vi "Testing FXP18-to-I16 conversions.vi"() -> ()   [LabVIEW 2015]
uses:
  <instrlib>/_niInstr/DSP/v1/Shared/Public/IQ Data.ctl
  DDC_7976R_v1.lvlib
  <vilib>/Analysis/NI_AALBase.lvlib
  <instrlib>/_niInstr/DSP/v1/Shared/niInstr DSP v1 Shared.lvlib
panel:
  out "appended array":dbl[][](graph)
  out "double precision float":dbl
  out "*(type *) &x":fxp<+/-,18,1> format="%.18g"
  out "Numeric Control":u32
  in  "data":T1
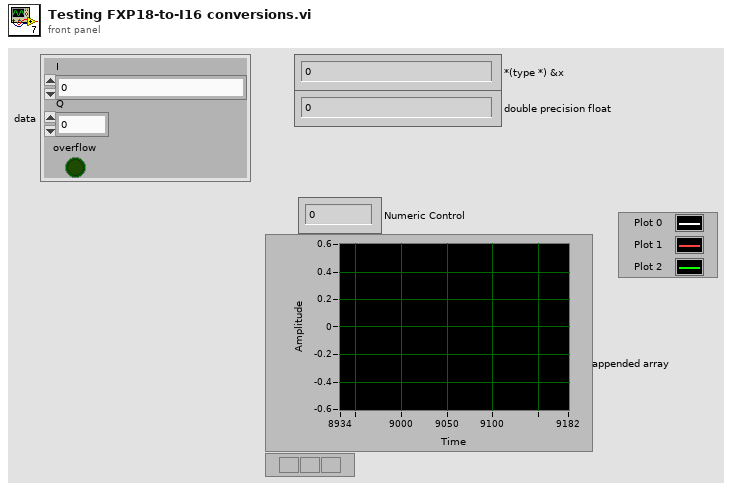
[diagram p1: front panel]
types:
  T1 = typedef "niInstr DSP v1 Shared.lvlib/IQ Data.ctl" = cluster{"I":fxp<+/-,18,1>, "Q":fxp<+/-,18,1>, "overflow":bool}
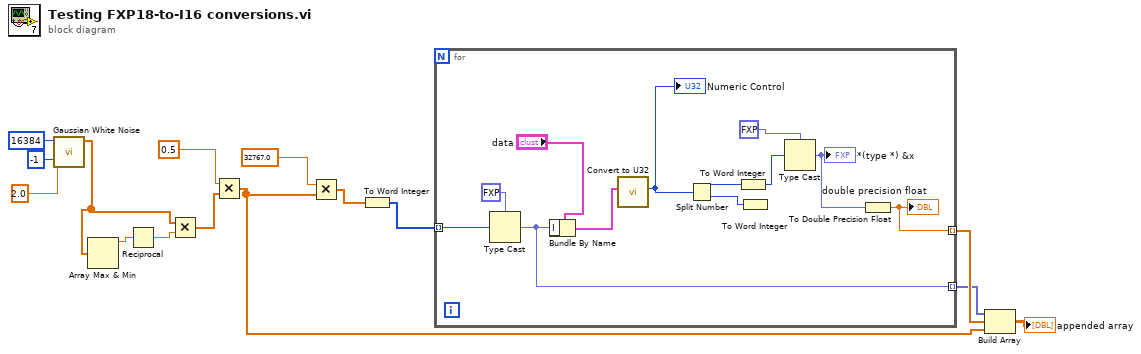
[diagram p0: block diagram]
diagram:
  n1 = call <vilib>:"Gaussian White Noise.vi"("seed"=-1, "standard deviation"=2.0, "samples"=16384) -> ("Gaussian noise pattern"=w7:dbl[])  [unwired: 7 in, 1 out]
  n2 = Array Max & Min(array=w7) -> (max value=w8:dbl)  [unwired: 3 out]
  n3 = Reciprocal(x=w8) -> (1/x=w6:dbl)
  n4 = Multiply(x=w7, y=w6) -> (x*y=w5:dbl[])
  n5 = Multiply(x=0.5, y=w5) -> (x*y=w3:dbl[])
  n6 = Multiply(x=32767.0, y=w3) -> (x*y=w1:dbl[])
  n7 = To Word Integer(number=w1) -> (16bit integer=w4:i16[])
  n8 = for {
    tunnel: w4 -> [w19] mode=indexing
    tunnel: [w18] -> w14 mode=indexing
    tunnel: [w16] -> w12 mode=indexing
    n9 = Type Cast(type=fxp<+/-,18,1> 0.0 ("I"), x=w19) -> (*(type *) &x=w16:fxp<+/-,18,1>)
    n10 = Bundle By Name(cluster="data", "I"=w16) -> (w17:T1)
    n11 = call "Convert to U32.vi"("data"=w17) -> ("Numeric Control"=w27:u32)  [unwired: 9 in, 1 out]
    "Numeric Control" <- w27
    n12 = Split Number(x=w27) -> (hi(x)=w26:u16, lo(x)=w25:u16)
    n13 = To Word Integer(number=w26) -> (16bit integer=w24:i16)
    n14 = To Word Integer(number=w25) -> ()  [unwired: 1 out]
    n15 = Type Cast(type=fxp<+/-,18,1> 0.0 ("I"), x=w24) -> (*(type *) &x=w22:fxp<+/-,18,1>)
    "*(type *) &x" <- w22
    n16 = To Double Precision Float(number=w22) -> (double precision float=w18:dbl)
    "double precision float" <- w18
  }
  n17 = Build Array(w12, w14, w3) -> (→"appended array":dbl[][])
